vi "Joy1Buttons.vi"() -> ()   [LabVIEW 2018]
panel:
  out "Left":bool
  out "Right":bool
  out "Down":bool
  out "Up":bool
  in  "Left Button":bool
  in  "Right Button":bool
  in  "Button Y":bool
  in  "Button X":bool
  in  "Button B":bool
  in  "Button A":bool
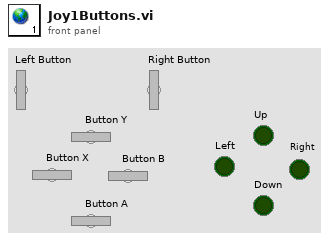
[diagram p1: front panel]
diagram:
